vi "3.1.1-VectorNav_Test.vi"() -> ()   [LabVIEW 2010]
uses:
  <vilib>/rvi/interface/nirviMethod/nirviMethod.xnode
  <vilib>/rvi/interface/nirviOpenFPGA/nirviOpenFPGA.xnode
  <vilib>/userDefined/High Color/nirio_resource_hc.ctl
  <vilib>/Utility/error.llb/Error Cluster From Error Code.vi
  <vilib>/rvi/interface/nirviCloseFPGA/nirviCloseFPGA.xnode
  NiFpgaLv.dll
  <vilib>/FPGAPlugInAG/Dynamic/niLvFpga_Close_Dynamic.vi
  <vilib>/rvi/errors/niLvFpgaWhatHappensToTopLevelVI.ctl
  <vilib>/rvi/interface/common/niFpgaNodeNameForErrorReporting.ctl
  <vilib>/rvi/errors/niLvFpgaAdjustHostInterfaceError.vi
  FPGA Bitfiles/DaveBrain_FPGATarget_1.2.1-VectorNavR_8EA85E47.lvbitx
  1-Hindbrain/1.2-Where/1.2.1-VectorNav/1.2.1-VectorNav Read Write.vi
  <vilib>/FPGAPlugInAG/cRIO-9104/niLvFpga_Open_cRIO-9104.vi
  <vilib>/rvi/ClientSDK/nirviWhatTheDeviceIsDoing.ctl
  <vilib>/rvi/interface/common/dynamic/niFpgaDynamicAddResources.vi
panel:
  out "string":string
  out "Elements Remaining":u32
  in  "stop":bool
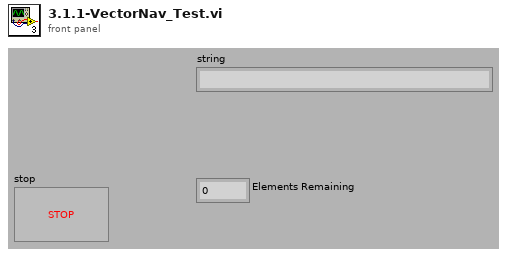
[diagram p1: front panel]
types:
  T1 = typedef "niFpgaNodeNameForErrorReporting.ctl" = enum16{"Open FPGA VI Reference", "Read/Write Control", "Invoke Method: Abort", "Invoke Method: Acknowledge IRQ", "Invoke Method: Download", "Invoke Method: FIFO.Configure", "Invoke Method: FIFO.Read", "Invoke Method: FIFO.Start", "Invoke Method: FIFO.Stop", "Invoke Method: FIFO.Write", "Invoke Method: Reset", "Invoke Method: Run", "Invoke Method: Wait on IRQ", "Close FPGA VI Reference"}
  T2 = typedef "niLvFpgaWhatHappensToTopLevelVI.ctl" = enum16{"top level VI scripted behind XNode", "top level VI inlined behind XNode"}
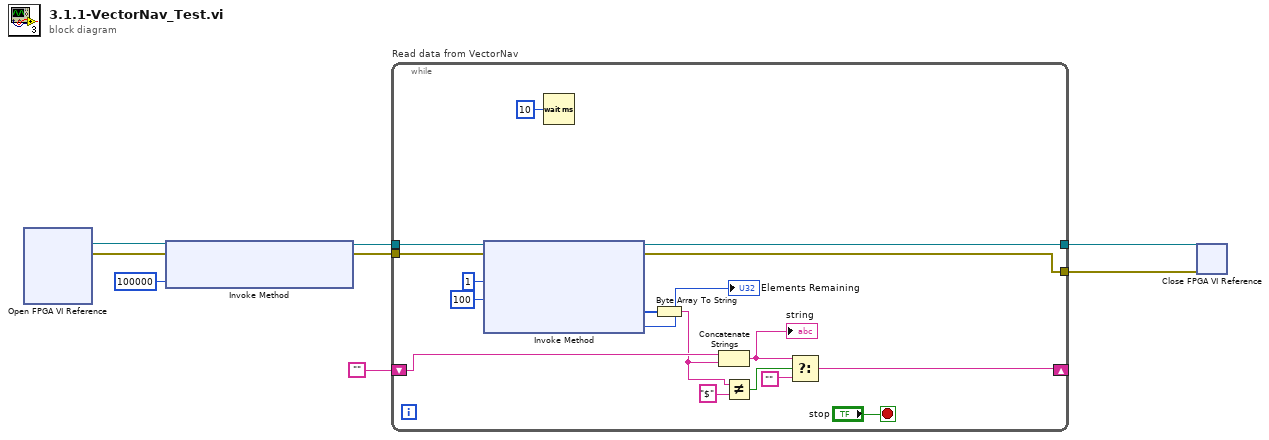
[diagram p0: block diagram]
diagram:
  n1 = xnode "Open FPGA VI Reference"() -> ("FPGA VI Reference Out"=w7:refnum<k20>, "error out"=w8:errorcluster)  [unwired: 2 in]
  n2 = xnode "Invoke Method"("FPGA VI Reference In"=w7, "error in"=w8, "Depth"=u32 100000) -> ("FPGA VI Reference Out"=w5:refnum<k20>, "error out"=w4:errorcluster)
  n3 = while "Read data from VectorNav" {
    tunnel: w5 -> [w25]
    tunnel: w4 -> [w24]
    tunnel: [w21] -> w3
    tunnel: [w20] -> w2
    shift-right: [w11] -> _
    shift-left: "" -> [w17]
    stop <- "stop" stop-if-true
    n4 = xnode "Invoke Method"("FPGA VI Reference In"=w25, "error in"=w24, "Number of Elements"=u32 1, "Timeout (ms)"=100) -> ("FPGA VI Reference Out"=w21:refnum<k20>, "error out"=w20:errorcluster, "Data"=w19:u8[], "Elements Remaining"=→"Elements Remaining":u32)
    n5 = Wait (ms)(milliseconds to wait=u32 10) -> ()  [unwired: 1 out]
    n6 = Byte Array To String(unsigned byte array=w19) -> (string=w14:string)
    n7 = Concatenate Strings(w17, w14) -> (w15:string)
    "string" <- w15
    n8 = Not Equal?(x=w14, y="$") -> (x != y?=w12:bool)
    n9 = Select(t=w15, s=w12, f="") -> (s? t:f=w11:string)
  }
  n10 = xnode "Close FPGA VI Reference"("FPGA VI Reference In"=w3, "error in"=w2) -> ()  [unwired: 1 out]
